vi "FaulhaberV3-Ascii_V1.vi"() -> (1 "searchnames":string[](array[string])=["devicetype", "errorregister", "pre-definederrorfield_numberoferrors", "pre-definederrorfield_standarderrorfield1", "pre-definederrorfield_standarderrorfield2", "pre-definederrorfield_standarderrorfield3", "pre-definederrorfield_standarderrorfield4", "pre-definederrorfield_standarderrorfield5", "pre-definederrorfield_standarderrorfield6", "pre-definederrorfield_standarderrorfield7", "pre-definederrorfield_standarderrorfield8", "cob-idsync", "manufacturerdevicename", "manufacturerhardwareversion", "manufacturersoftwareversion", "guardtime", "lifetimefactor", "storeparameters_numberofentries", "storeparameters_saveallparameters", "storeparameters_savecommparameters", "storeparameters_saveappparameters", "storeparameters_saveappparameters1", "storeparameters_saveappparameters2", "storeparameters_savecalparameters", "storeparameters_savefactoryparameteralls", "storeparameters_savefactoryparameterscom", "storeparameters_savefactoryparametersapp", "restoredefaultparameters_numberofentries", "restoredefaultparameters_restorealldefaultparameters", "restoredefaultparameters_restorecommdefaultparameters", "restoredefaultparameters_restoreappdefaultparameters", "restoredefaultparameters_restoreappsaved", "restoredefaultparameters_restoreapp1saved", "restoredefaultparameters_restoreapp2saved", "cob-idemcy", "consumerheartbeattime_numberofentries", "consumerheartbeattime_consumerheartbeattime", "producerheartbeattime", "identityobject_numberofentries", "identityobject_vendorid", "identityobject_productcode", "identityobject_revisionnumber", "identityobject_serialnumber", "errorbehaviour/numberoferrorclasses_numberoferrorclasses", "errorbehaviour/numberoferrorclasses_communicationerror", "serversdoparameter_numberofentries", "serversdoparameter_cob-idclienttoserver(rx)", "serversdoparameter_cob-idservertoclient(tx)", "receivepdo1parameter_numberofentries", "receivepdo1parameter_cob-idusedbyrxpdo1", "receivepdo1parameter_transmissiontype", "receivepdo2parameter_numberofentries", "receivepdo2parameter_cob-idusedbyrxpdo2", "receivepdo2parameter_transmissiontype", "receivepdo3parameters_numberofentries", "receivepdo3parameters_cob-idusedbyrxpdo3", "receivepdo3parameters_transmissiontype", "receivepdo4parameter_numberofentries", "receivepdo4parameter_cob-idusedbyrxpdo4", "receivepdo4parameter_transmissiontype", "receivepdo1mapping/numberofmappedobjects_numberofmappedobjects", "receivepdo1mapping/numberofmappedobjects_rxpdo1mappingentry1", "receivepdo1mapping/numberofmappedobjects_rxpdo1mappingentry2", "receivepdo1mapping/numberofmappedobjects_rxpdo1mappingentry3", "receivepdo1mapping/numberofmappedobjects_rxpdo1mappingentry4", "receivepdo2mapping/numberofmappedobjects_numberofmappedobjects", "receivepdo2mapping/numberofmappedobjects_rxpdo2mappingentry1", "receivepdo2mapping/numberofmappedobjects_rxpdo2mappingentry2", "receivepdo2mapping/numberofmappedobjects_rxpdo2mappingentry3", "receivepdo2mapping/numberofmappedobjects_rxpdo2mappingentry4", "receivepdo3mapping/numberofmappedobjects_numberofmappedobjects", "receivepdo3mapping/numberofmappedobjects_rxpdo3mappingentry1", "receivepdo3mapping/numberofmappedobjects_rxpdo3mappingentry2", "receivepdo3mapping/numberofmappedobjects_rxpdo3mappingentry3", "receivepdo3mapping/numberofmappedobjects_rxpdo3mappingentry4", "receivepdo4mapping/numberofmappedobjects_numberofmappedobjects", "receivepdo4mapping/numberofmappedobjects_rxpdo4mappingentry1", "receivepdo4mapping/numberofmappedobjects_rxpdo4mappingentry2", "receivepdo4mapping/numberofmappedobjects_rxpdo4mappingentry3", "receivepdo4mapping/numberofmappedobjects_rxpdo4mappingentry4", "transmitpdo1parameter_numberofentries", "transmitpdo1parameter_cob-idusedbytxpdo1", "transmitpdo1parameter_transmissiontype", "transmitpdo1parameter_eventtimer", "transmitpdo2parameter_numberofentries", "transmitpdo2parameter_cob-idusedbytxpdo2", "transmitpdo2parameter_transmissiontype", "transmitpdo2parameter_eventtimer", "transmitpdo3parameter_numberofentries", "transmitpdo3parameter_cob-idusedbytxpdo3", "transmitpdo3parameter_transmissiontype", "transmitpdo3parameter_eventtimer", "transmitpdo4parameter_numberofentries", "transmitpdo4parameter_cob-idusedbytxpdo4", "transmitpdo4parameter_transmissiontype", "transmitpdo4parameter_eventtimer", "transmitpdo1mapping/numberofmappedobjects_numberofmappedobjects", "transmitpdo1mapping/numberofmappedobjects_tpdo1mappingentry1", "transmitpdo1mapping/numberofmappedobjects_tpdo1mappingentry2", "transmitpdo1mapping/numberofmappedobjects_txpdo1mappingentry3", "transmitpdo1mapping/numberofmappedobjects_txpdo1mappingentry4", "transmitpdo2mapping/numberofmappedobjects_numberofmappedobjects", "transmitpdo2mapping/numberofmappedobjects_txpdo1mappingentry1", "transmitpdo2mapping/numberofmappedobjects_txpdo2mappingentry2", "transmitpdo2mapping/numberofmappedobjects_txpdo3mappingentry3", "transmitpdo2mapping/numberofmappedobjects_txpdo4mappingentry4", "transmitpdo3mapping/numberofmappedobjects_numberofmappedobjects", "transmitpdo3mapping/numberofmappedobjects_txpdo3mappingentry1", "transmitpdo3mapping/numberofmappedobjects_txpdo3mappingentry2", "transmitpdo3mapping/numberofmappedobjects_txpdo3mappingentry3", "transmitpdo3mapping/numberofmappedobjects_txpdo3mappingentry4", "transmitpdo4mapping/numberofmappedobjects_numberofmappedobjects", "transmitpdo4mapping/numberofmappedobjects_txpdo4mappingentry1", "transmitpdo4mapping/numberofmappedobjects_txpdo4mappingentry2", "transmitpdo4mapping/numberofmappedobjects_txpdo4mappingentry3", "transmitpdo4mapping/numberofmappedobjects_txpdo4mappingentry4", "numberofi/os_numberofentries", "numberofi/os_numberofdigitalinputs", "numberofi/os_numberofdigitaloutputs", "numberofi/os_numberofanaloginputs", "numberofi/os_numberofemulateddigitalinputs", "digitalinputsettings_numberofentries", "digitalinputsettings_selectlowerlimitswitchinputs", "digitalinputsettings_selectupperlimitswitchinputs", "digitalinputsettings_limitswitchoptioncode", "digitalinputsettings_selectreferenceswitchinput", "digitalinputsettings_emulatedinputthresholdlevel", "digitalinputsettings_selectstopinput", "digitalinputsettings_debugwritedigitalinputvalues", "digitalinputsettings_debugwritebrake/faultpin", "digitalinputsettings_selectdigitalinputsused", "digitalinputsettings_inputpolarity", "digitalinputsettings_inputthresholdlevel", "digitalinputsettings_inputfilteractive", "digitali/ostatus_numberofentries", "digitali/ostatus_digitalinputlogicalstate", "digitali/ostatus_digitalinputphysicalstate", "digitali/ostatus_digitaloutputstatus", "digitali/ostatus_writedigitaloutputs", "digitaloutputsettings_numberofentries", "digitaloutputsettings_selectfaultoutputpin", "digitaloutputsettings_selectbrakecontrolpin", "digitaloutputsettings_brakedelaytime", "digitaloutputsettings_diagout1pinselection", "digitaloutputsettings_diagout1mask", "digitaloutputsettings_diagout2pinselection", "digitaloutputsettings_diagout2mask", "digitaloutputsettings_diagout3pinselection", "digitaloutputsettings_diagout3mask", "digitaloutputsettings_diagout4pinselection", "digitaloutputsettings_diagout4mask", "digitaloutputsettings_outputpolarity", "analoginputs_numberofentries", "analoginputs_anin1gain(numerator/divisor)", "analoginputs_anin1offset", "analoginputs_anin1filtertime", "analoginputs_anin1userscaledvalue", "analoginputs_anin1resolutionasencoder", "analoginputs_anin1mininputlimit", "analoginputs_anin1maxinputlimit", "analoginputs_anin1selectdirpin", "analoginputs_anin1virtualinputvalue", "analoginputs_anin1enablevirtualinput", "analoginputs_anin2gain(numerator/divisor)", "analoginputs_anin2offset", "analoginputs_anin2filtertime", "analoginputs_anin2userscaledvalue", "analoginputs_anin2resolutionasencoder", "analoginputs_anin2mininputlimit", "analoginputs_anin2maxinputlimit", "analoginputs_anin2selectdirpin", "analoginputs_anin2virtualinputvalue", "analoginputs_anin2enablevirtualinput", "manufacturerscaledanaloginputvalues_numberofentries", "manufacturerscaledanaloginputvalues_anin1scaledvalue(ia)", "manufacturerscaledanaloginputvalues_anin2scaledvalue(ib)", "manufacturerscaledanaloginputvalues_anin3scaledvalue(ic)", "manufacturerscaledanaloginputvalues_anin4scaledvalue(halla)", "manufacturerscaledanaloginputvalues_anin5scaledvalue(hallb)", "manufacturerscaledanaloginputvalues_anin6scaledvalue(hallc)", "manufacturerscaledanaloginputvalues_anin7scaledvalue", "manufacturerscaledanaloginputvalues_anin8scaledvalue", "manufacturerscaledanaloginputvalues_anin9scaledvalue", "manufacturerscaledanaloginputvalues_anin10scaledvalue", "manufacturerscaledanaloginputvalues_anin11scaledvalue", "manufacturerscaledanaloginputvalues_anin12scaledvalue", "motorencoder_numberofentries", "motorencoder_operationmode,indexpolarity", "motorencoder_ieresolution", "motorencoder_motorencoderposition", "motorencoder_gain(numerator/divisor)", "motorencoder_motorencscaledposition", "motorencoder_absoluteencoderbits", "motorencoder_encoderstatus", "motorencoder_motorencoderactspeed", "motorencoder_speedfilter", "motorencoder_singleturnposition16bit", "referenceencoder_numberofentries", "referenceencoder_operationmode,indexpolarity", "referenceencoder_ieresolution", "referenceencoder_referenceencoderposition", "referenceencoder_gain(numerator/divisor)", "referenceencoder_refencscaledposition", "referenceencoder_referenceencoderactspeed", "referenceencoder_speedfilter", "pwminput_numberofentries", "pwminput_digitalinputpin", "pwminput_pwminputfrequency", "pwminput_dutycyclerawvalue", "pwminput_dutycyclegain(numerator/divisor)", "pwminput_dutycycleoffset", "pwminput_dutycyclescaledvalue", "pwminput_resolutionasencoder", "hallconfiguration_numberofentries", "hallconfiguration_hallsensortype", "hallconfiguration_enableadaptation", "hallconfiguration_adaptationthresholdspeed", "hallconfiguration_digitalhallsettingsofnon-faulhabermotors", "hallconfiguration_hallfilterconfiguration", "reductionratio,externalpositionencoder_numberofentries", "reductionratio,externalpositionencoder_numerator", "reductionratio,externalpositionencoder_divisor", "231f_00_numberofentries", "231f_00_231f_01", "231f_00_231f_02", "231f_00_231f_03", "231f_00_231f_04", "231f_00_231f_05", "231f_00_231f_06", "231f_00_231f_07", "231f_00_231f_08", "231f_00_231f_09", "231f_00_231f_0a", "231f_00_231f_0b", "231f_00_231f_0c", "231f_00_231f_0d", "231f_00_231f_0e", "231f_00_231f_0f", "faulhabererrorregister", "errormask_numberofentries", "errormask_emcymask", "errormask_faultmask", "errormask_erroroutmask", "errormask_disablevoltagemaskmanufacturer", "errormask_disablevoltagemaskuser", "errormask_quickstopmask", "errormask_errorbitmask", "errorcodes_numberofentries", "errorcodes_scriptingerror", "devicestatus_numberofentries", "devicestatus_devicestatusword", "devicestatus_limitcheckdelaytime", "devicestatus_reserved3", "devicestatus_reserved4", "devicestatus_reserved5", "devicestatus_reserved6", "devicestatus_reserved7", "devicestatus_reserved8", "devicestatus_reserved9", "voltagemonitor_numberofentries", "voltagemonitor_devicesupplylowerthreshold", "voltagemonitor_motorsupplylowerthreshold", "voltagemonitor_motorsupplymaxthreshold", "voltagemonitor_motorsupplyupperthreshold", "voltagemonitor_voltageerrordelaytime", "voltagemonitor_devicesupplyvoltage", "voltagemonitor_motorsupplyvoltage", "devicetemperature_numberofentries", "devicetemperature_cputemperature", "devicetemperature_powerstagetemperature", "devicetemperature_windingtemperature", "devicetemperature_cputemperatureshutdownthreshold", "devicetemperature_cputemperaturewarningthreshold", "devicetemperature_powerstagetemperatureshutdownthreshold", "devicetemperature_powerstagetemperaturewarningthreshold", "devicetemperature_windingtemperatureshutdownthreshold", "devicetemperature_windingtemperaturewarningthreshold", "devicetemperature_motorntctemperature", "devicetemperature_motorntcenable", "devicedata_numberofentries", "devicedata_devicenominalcurrent", "devicedata_devicepeakcurrent", "devicedata_devicenominalvoltage", "devicedataforthermalmodel_numberofentries", "devicedataforthermalmodel_controllertype", "devicedataforthermalmodel_powerstagerdson", "devicedataforthermalmodel_powerstagelossfactor", "devicedataforthermalmodel_powerstagerth1", "devicedataforthermalmodel_powerstagetimeconstant1", "devicedataforthermalmodel_powerstagerth2", "devicedataforthermalmodel_powerstagetimeconstant2", "devicedataforthermalmodel_powerstagerth3", "devicedataforthermalmodel_powerstagerth4", "motorandapplicationdataformotorcontrol_numberofentries", "motorandapplicationdataformotorcontrol_ratedcurrent", "motorandapplicationdataformotorcontrol_continouscurrent", "motorandapplicationdataformotorcontrol_peakcurrent", "motorandapplicationdataformotorcontrol_torqueconstant/forceconstant", "motorandapplicationdataformotorcontrol_terminalinductance", "motorandapplicationdataformotorcontrol_inductanceld", "motorandapplicationdataformotorcontrol_numberofpolepairs", "motorandapplicationdataformotorcontrol_phaseangleoffset", "motorandapplicationdataformotorcontrol_rotorinertia/rodweight", "motorandapplicationdataformotorcontrol_loadinertia/loadmass", "motorandapplicationdataformotorcontrol_motortype", "motorandapplicationdataformotorcontrol_magneticpitchoflinearmotor", "motorandapplicationdataformotorcontrol_filterphaseinductance", "motorandapplicationdataformotorcontrol_factorspeedconstant", "motorandapplicationdataformotorcontrol_stepsperturn", "motorandapplicationdataformotorcontrol_stepperinterpolationfactor", "motorandapplicationdataformotorcontrol_steppercurrentreductionatn=0", "motorandapplicationdataformotorcontrol_currentholdingtimeatn=0", "motorandapplicationdataforthermalmotormodel_numberofentries", "motorandapplicationdataforthermalmotormodel_terminalresistance", "motorandapplicationdataforthermalmotormodel_friction", "motorandapplicationdataforthermalmotormodel_friction,dynamic", "motorandapplicationdataforthermalmotormodel_thermalresistance1", "motorandapplicationdataforthermalmotormodel_thermalresistance2", "motorandapplicationdataforthermalmotormodel_thermaltimeconstant1", "motorandapplicationdataforthermalmotormodel_thermaltimeconstant2", "motorandapplicationdataforthermalmotormodel_ambienttemperature", "motorandapplicationdataforthermalmotormodel_reductionofthermalresistance2", "motorandapplicationdataforthermalmotormodel_selectionofthermalmodel", "motoralignmentparameters_numberofentries", "motoralignmentparameters_setuptime", "motoralignmentparameters_deltatimestep1", "motoralignmentparameters_deltatimestep2", "motoralignmentparameters_deltatimestep3", "motoralignmentparameters_deltapostiontolerance", "motoralignmentresults_numberofentries", "motoralignmentresults_positiona1", "motoralignmentresults_positionb", "motoralignmentresults_positiona2", "switchpositionforactualvalues_numberofentries", "switchpositionforactualvalues_actualcommutationanglesource", "switchpositionforactualvalues_actualvelocitysource", "switchpositionforactualvalues_actualpositionsource", "discretesources_numberofentries", "discretesources_targetvoltagesource", "discretesources_targetcurrentsource", "discretesources_targetvelocitysource", "discretesources_targetpositionsource", "cyclicmodeinterpolationrate", "manufacturerspecifiedbits_numberofentries", "manufacturerspecifiedbits_bitmaskforbit14", "manufacturerspecifiedbits_bitmaskforbit15", "selectionofcontrollerscaling", "operationmodeoptions", "generalparameters_numberofentries", "generalparameters_commutationtype", "generalparameters_motoroutputvoltagedc", "generalparameters_motoroutputvoltageblblock", "generalparameters_motoroutputvoltagexd", "generalparameters_motoroutputvoltagexq", "generalparameters_sinusoutputvoltageua", "generalparameters_sinusoutputvoltageub", "generalparameters_sinusoutputvoltageuc", "generalparameters_sinusoutputvoltageud", "targetvoltage", "torquecontrolparameters_numberofentries", "torquecontrolparameters_gainkpi", "torquecontrolparameters_integraltimetni", "fluxcontrolparameters_numberofentries", "fluxcontrolparameters_gainkpi", "fluxcontrolparameters_integraltimetni", "velocitycontrolparameters_numberofentries", "velocitycontrolparameters_gainkp", "velocitycontrolparameters_integraltimetn", "velocitycontrolparameters_velocitydeviationthreshold", "velocitycontrolparameters_velocitydeviationtime", "velocitycontrolparameters_velocitywarningthreshold", "velocitycontrolparameters_integralpartoption", "velocityfilterparameters_numberofentries", "velocityfilterparameters_actualvelocityfiltertf", "velocityfilterparameters_displayvelocityfilter", "setpointvelocityfilterparameters_numberofentries", "setpointvelocityfilterparameters_setpointvelocityfiltertf", "setpointvelocityfilterparameters_setpointfilterenable", "gainscheduling_numberofentries", "gainscheduling_gainfactorkpn", "gainscheduling_gainfactorkv", "positioncontrolparameters_numberofentries", "positioncontrolparameters_gainkv", "currentfeedforwardparameters_numberofentries", "currentfeedforwardparameters_currentfeedforwardfactor", "currentfeedforwardparameters_currentfeedforwarddelay", "velocityfeedforwardparameters_numberofentries", "velocityfeedforwardparameters_velocityfeedforwardfactor", "velocityfeedforwardparameters_velocityfeedforwarddelay", "currentfilterparameters_numberofentries", "currentfilterparameters_displaycurrentfiltertf", "currentfilterparameters_displaytorquefiltertf", "currentcompensationparameters_numberofentries", "currentcompensationparameters_gravitycompensation", "currentcompensationparameters_positivefrictioncompensation", "currentcompensationparameters_negativefrictioncompensation", "positivetorquelimithoming", "negativetorquelimithoming", "actualvalues_numberofentries", "actualvalues_motorcurrentidactualvalue", "actualvalues_motorcurrentiqactualvalue", "actualvalues_motorcurrrentiblockactualvalue", "actualvalues_motorcurrentidcactualvalue", "actualvalues_velocityactualinternalvalue", "actualvalues_positionactualinternalvalue", "actualvalues_actualcommutationsegment", "actualvalues_actualcommutationangle", "actualvalues_reserved9", "actualvalues_reserved10", "traceconfiguration_numberofentries", "traceconfiguration_triggervalue", "traceconfiguration_triggerthreshold", "traceconfiguration_triggeroffset", "traceconfiguration_triggermode", "traceconfiguration_bufferlength", "traceconfiguration_sampletime", "traceconfiguration_tracesourceofchannel1", "traceconfiguration_tracesourceofchannel2", "traceconfiguration_tracesourceofchannel3", "traceconfiguration_tracesourceofchannel4", "traceconfiguration_monitorsourceofchannel1", "traceconfiguration_monitorsourceofchannel2", "traceconfiguration_monitorsourceofchannel3", "traceconfiguration_monitorsourceofchannel4", "traceconfiguration_extendedrecordermode", "tracebuffer_numberofentries", "tracebuffer_tracestate", "logictriggerconfiguration_numberofentries", "logictriggerconfiguration_logictriggerandmask", "logictriggerconfiguration_logictriggerormask", "eventtriggerconfiguration_numberofentries", "eventtriggerconfiguration_eventtriggereventselection", "eventflagconfiguration_numberofentries", "eventflagconfiguration_eventflagsetmask", "eventflagconfiguration_eventflagresetmask", "tracechannelconfiguration_numberofentries", "tracechannelconfiguration_channel1filtertime", "tracechannelconfiguration_channel1sampletime", "tracechannelconfiguration_channel1numberofsamples", "tracechannelconfiguration_channel1monitoringvalues", "tracechannelconfiguration_channel1starteventselection", "tracechannelconfiguration_channel1updateeventselection", "tracechannelconfiguration_channel1numberofeval-cycles", "tracechannelconfiguration_channel1numberofturnovers", "tracechannelconfiguration_channel1done", "tracechannelconfiguration_channel1absminvalue", "tracechannelconfiguration_channel1absmaxvalue", "tracechannelconfiguration_channel1minimum", "tracechannelconfiguration_channel1maximum", "tracechannelconfiguration_channel1meanvalue", "tracechannelconfiguration_channel1rmsvalue", "tracechannelconfiguration_channel1periodtime", "tracechannelconfiguration_channel1sigma", "tracechannelconfiguration_numberofentries", "tracechannelconfiguration_channel2filtertime", "tracechannelconfiguration_channel2sampletime", "tracechannelconfiguration_channel2numberofsamples", "tracechannelconfiguration_channel2monitoringvalues", "tracechannelconfiguration_channel2starteventselection", "tracechannelconfiguration_channel2updateeventselection", "tracechannelconfiguration_channel2numberofeval-cycles", "tracechannelconfiguration_channel2numberofturn-overs", "tracechannelconfiguration_channel2done", "tracechannelconfiguration_channel2absminvalue", "tracechannelconfiguration_channel2absmaxvalue", "tracechannelconfiguration_channel2minimum", "tracechannelconfiguration_channel2maximum", "tracechannelconfiguration_channel2meanvalue", "tracechannelconfiguration_channel2rmsvalue", "tracechannelconfiguration_channel2periodtime", "tracechannelconfiguration_channel2sigma", "tracechannelconfiguration_numberofentries", "tracechannelconfiguration_channel3filtertime", "tracechannelconfiguration_channel3sampletime", "tracechannelconfiguration_channel3numberofsamples", "tracechannelconfiguration_channel3monitoringvalues", "tracechannelconfiguration_channel3starteventselection", "tracechannelconfiguration_channel3updateeventselection", "tracechannelconfiguration_channel3numberofeval-cycles", "tracechannelconfiguration_channel3numberofturn-overs", "tracechannelconfiguration_channel3done", "tracechannelconfiguration_channel3absminvalue", "tracechannelconfiguration_channel3absmaxvalue", "tracechannelconfiguration_channel3minimum", "tracechannelconfiguration_channel3maximum", "tracechannelconfiguration_channel3meanvalue", "tracechannelconfiguration_channel3rmsvalue", "tracechannelconfiguration_channel3periodtime", "tracechannelconfiguration_channel3sigma", "tracechannelconfiguration_numberofentries", "tracechannelconfiguration_channel4filtertime", "tracechannelconfiguration_channel4sampletime", "tracechannelconfiguration_channel4numberofsamples", "tracechannelconfiguration_channel4monitoringvalues", "tracechannelconfiguration_channel4starteventselection", "tracechannelconfiguration_channel4updateeventselection", "tracechannelconfiguration_channel4numberofeval-cycles", "tracechannelconfiguration_channel4numberofturn-overs", "tracechannelconfiguration_channel4done", "tracechannelconfiguration_channel4absminvalue", "tracechannelconfiguration_channel4absmaxvalue", "tracechannelconfiguration_channel4minimum", "tracechannelconfiguration_channel4maximum", "tracechannelconfiguration_channel4meanvalue", "tracechannelconfiguration_channel4rmsvalue", "tracechannelconfiguration_channel4periodtime", "tracechannelconfiguration_channel4sigma", "prbsgenerator_numberofentries", "prbsgenerator_shiftregisterinit", "prbsgenerator_gain", "prbsgenerator_offset", "prbsgenerator_sampleratefactor", "prbsgenerator_enable", "startupgenerator_numberofentries", "startupgenerator_speedthreshold", "startupgenerator_timeouttime", "startupgenerator_targetvalue", "startupgenerator_reset", "startupgenerator_enable", "startupgenerator_ready", "startupgenerator_timethreshold", "startupgenerator_iteration", "sinusoidalexcitation_numberofentries", "sinusoidalexcitation_amplitude", "sinusoidalexcitation_frequency", "sinusoidalexcitation_enable", "selectsignalgeneratorsource_numberofentries", "selectsignalgeneratorsource_selector", "23f0_00_numberofentries", "23f0_00_23f0_01", "23f0_00_23f0_02", "23f0_00_23f0_03", "23f0_00_23f0_04", "23f0_00_23f0_05", "23f0_00_23f0_06", "23f1_00_numberofentries", "23f1_00_23f1_01", "23f1_00_23f1_02", "23f2_00_numberofentries", "23f2_00_actualstate", "23f2_00_demandposition", "23f2_00_demandspeed", "23f2_00_demandacceleration", "23f2_00_initialstate", "communicationparameters_numberofentries", "communicationparameters_canrate", "communicationparameters_rs232rate", "communicationparameters_nodeid", "communicationparameters_communicationsettings", "communicationparameters_rs232netmode", "communicationparameters_comstate", "communicationparameters_errstate", "usbdelay", "faid", "bootloaderswversion", "odrevisionnumber", "swrevisionnumber", "xdcnumber", "calaccess_numberofentries", "calaccess_calkey", "adcscaling(offset|gain)_numberofentries", "adcscaling(offset|gain)_iascaling", "adcscaling(offset|gain)_ibscaling", "adcscaling(offset|gain)_icscaling", "adcscaling(offset|gain)_hallascaling", "adcscaling(offset|gain)_hallbscaling", "adcscaling(offset|gain)_hallcscaling", "adcscaling(offset|gain)_analoginput1scaling", "adcscaling(offset|gain)_analoginput2scaling", "adcscaling(offset|gain)_uelscaling", "adcscaling(offset|gain)_udcscaling", "adcscaling(offset|gain)_internaltemperaturescaling", "adcscaling(offset|gain)_externaltemperaturescaling", "adcscaling(offset|gain)_motorntcgain", "adcscaling(offset|gain)_motorntcoffset", "hallscaling_numberofentries", "hallscaling_gaina", "hallscaling_hallaoffset", "hallscaling_hallasin", "hallscaling_hallacos", "hallscaling_corra", "hallscaling_hallboffset", "hallscaling_hallbsin", "hallscaling_hallbcos", "hallscaling_corrb", "hallscaling_hallcoffset", "hallscaling_hallcsin", "hallscaling_hallccos", "hallscaling_offseta", "hallscaling_offsetb", "internalfilterparameters_numberofentries", "internalfilterparameters_filtertimeactualvelocity", "internalfilterparameters_filtertimeia", "internalfilterparameters_filtertimeib", "internalfilterparameters_filtertimeic", "internalfilterparameters_filtertimeuel", "internalfilterparameters_filtertimeumot", "internalfilterparameters_additionalfiltertimeuel", "internalfilterparameters_additionalfiltertimeumot", "internalfilterparameters_filtertimeiqthermalmodel", "internalfilterparameters_filtertimeidthermalmodel", "internalfilterparameters_filtertimeimotthermalmodel", "internalfilterparameters_filtertimesetpointvoltagemodel", "internalfilterparameters_filtertimeelectricaltimeconstant", "bootoptions", "hallcompensation_numberofentries", "hallcompensation_entry01", "hallcompensation_entry02", "hallcompensation_entry03", "hallcompensation_entry04", "hallcompensation_entry05", "hallcompensation_entry06", "hallcompensation_entry07", "hallcompensation_entry08", "hallcompensation_entry09", "hallcompensation_entry10", "hallcompensation_entry11", "hallcompensation_entry12", "encodercompensation_numberofentries", "encodercompensation_value0", "encodercompensation_value1", "encodercompensation_value2", "encodercompensation_value3", "encodercompensation_value4", "encodercompensation_value5", "encodercompensation_value6", "encodercompensation_value7", "encodercompensation_value8", "encodercompensation_value9", "encodercompensation_value10", "encodercompensation_value11", "encodercompensation_value12", "encodercompensation_value13", "encodercompensation_value14", "encodercompensation_value15", "encodercompensation_value16", "encodercompensation_value17", "encodercompensation_value18", "encodercompensation_value19", "encodercompensation_value20", "encodercompensation_value21", "encodercompensation_value22", "encodercompensation_value23", "encodercompensation_value24", "encodercompensation_value25", "encodercompensation_value26", "encodercompensation_value27", "encodercompensation_value28", "encodercompensation_value29", "encodercompensation_value30", "encodercompensation_value31", "encodercompensation_value32", "encodercompensation_value33", "encodercompensation_value34", "encodercompensation_value35", "encodercompensation_value36", "encodercompensation_value37", "encodercompensation_value38", "encodercompensation_value39", "encodercompensation_value40", "encodercompensation_value41", "encodercompensation_value42", "encodercompensation_value43", "encodercompensation_value44", "encodercompensation_value45", "encodercompensation_value46", "encodercompensation_value47", "encodercompensation_value48", "encodercompensation_value49", "encodercompensation_value50", "encodercompensation_value51", "encodercompensation_value52", "encodercompensation_value53", "encodercompensation_value54", "encodercompensation_value55", "encodercompensation_value56", "encodercompensation_value57", "encodercompensation_value58", "encodercompensation_value59", "encodercompensation_value60", "encodercompensation_value61", "encodercompensation_value62", "encodercompensation_value63", "pwmfrequency", "250f_00", "drivesystemgear_numberofentries", "drivesystemgear_gearrationum", "drivesystemgear_gearratioden", "drivesystemloadtransmission_numberofentries", "drivesystemloadtransmission_loadtransmission", "drivesystemloadtransmission_loadtransmissionrationum", "drivesystemloadtransmission_loadtransmissionratioden", "drivesystemnumbers_numberofentries", "drivesystemnumbers_gearcatalognumber", "drivesystemnumbers_encodercatalogenumber", "drivesystemnumbers_drivecombinationnumber", "drivesystemunits_numberofentries", "drivesystemunits_unitreference", "drivesystemunits_unitnames", "nominalvoltage", "drivesystemsettings", "oemdevicedata_numberofentries", "oemdevicedata_oemproductdescriptor", "oemdevicedata_oemproductcode", "oemdevicedata_oemserialnumber", "userprograms_numberofentries", "userprograms_userprogram1startaddress", "userprograms_userprogram2startaddress", "userprograms_userprogram3startaddress", "userprograms_userprogram4startaddress", "userprograms_userprogram5startaddress", "userprograms_userprogram6startaddress", "userprograms_userprogram7startaddress", "userprograms_userprogram8startaddress", "activeprogram_numberofentries", "activeprogram_actualprogramcommand", "activeprogram_actualprogramnumber", "activeprogram_actualprogramposition", "activeprogram_actualprogramstate", "activeprogram_breakpointaddress", "activeprogram_upload/downloadbuffer", "activeprogram_errorstate", "activeprogram_errorcode", "activeprogram_programmemory", "autostartprogram", "accesskey", "debuguserprogram_numberofentries", "debuguserprogram_selectvariable", "debuguserprogram_selectedvariablevalue", "userprogramvariables_numberofentries", "userprogramvariables_userprogvariablea", "userprogramvariables_userprogvariableb", "userprogramvariables_userprogvariablec", "userprogramvariables_userprogvariabled", "userprogramvariables_userprogvariablee", "userprogramvariables_userprogvariablef", "userprogramvariables_userprogvariableg", "userprogramvariables_userprogvariableh", "userprogramvariables_userprogvariablei", "userprogramvariables_userprogvariablej", "userprogramvariables_userprogvariablek", "userprogramvariables_userprogvariablel", "userprogramvariables_userprogvariablem", "userprogramvariables_userprogvariablen", "userprogramvariables_userprogvariableo", "userprogramvariables_userprogvariablep", "userprogramvariables_userprogvariableq", "userprogramvariables_userprogvariabler", "userprogramvariables_userprogvariables", "userprogramvariables_userprogvariablet", "userprogramvariables_userprogvariableu", "userprogramvariables_userprogvariablev", "userprogramvariables_userprogvariablew", "userprogramvariables_userprogvariablex", "userprogramvariables_userprogvariabley", "userprogramvariables_userprogvariablez", "scriptingstack/numberoflevels_numberoflevels", "scriptingstack/numberoflevels_callstacklevel0", "scriptingstack/numberoflevels_callstacklevel1", "scriptingstack/numberoflevels_callstacklevel2", "scriptingstack/numberoflevels_callstacklevel3", "scriptingstack/numberoflevels_callstacklevel4", "scriptingstack/numberoflevels_callstacklevel5", "scriptingstack/numberoflevels_callstacklevel6", "scriptingstack/numberoflevels_callstacklevel7", "scriptingstack/numberoflevels_callstacklevel8", "scriptingstack/numberoflevels_callstacklevel9", "scriptingstack/numberoflevels_callstacklevel10", "scriptingstack/numberoflevels_callstacklevel11", "scriptingstack/numberoflevels_callstacklevel12", "scriptingstack/numberoflevels_callstacklevel13", "scriptingstack/numberoflevels_callstacklevel14", "variableaccesskey", "programconstants_numberofentries", "programconstants_programconstant0", "programconstants_programconstant1", "programconstants_programconstant2", "programconstants_programconstant3", "programconstants_programconstant4", "programconstants_programconstant5", "programconstants_programconstant6", "programconstants_programconstant7", "programconstants_programconstant8", "programconstants_programconstant9", "programconstants_programconstant10", "programconstants_programconstant11", "programconstants_programconstant12", "programconstants_programconstant13", "programconstants_programconstant14", "programconstants_programconstant15", "abortconnectionoptioncode", "controlword", "statusword", "quick-stopoptioncode", "shutdownoptioncode", "disableoperationoptioncode", "haltoptioncode", "faultreactionoptioncode", "modesofoperation", "modesofoperationdisplay", "positiondemandvalue", "positionactualinternalvalue", "positionactualvalue", "followingerrorwindow", "followingerrortimeout", "positionwindow", "positionwindowtime", "velocitydemandvalue", "velocityactualvalue", "velocitywindow", "velocitywindowtime", "velocitythreshold", "velocitythresholdtime", "targettorque", "maxtorque", "torquedemand", "torqueactualvalue", "currentactualvalue", "targetposition", "positionrangelimit_numberofentries", "positionrangelimit_minpositionrangelimit", "positionrangelimit_maxpositionrangelimit", "homeoffset", "softwarepositionlimit_numberofentries", "softwarepositionlimit_minpositionlimit", "softwarepositionlimit_maxpositionlimit", "polarity", "maxmotorspeed", "profilevelocity", "profileacceleration", "profiledeceleration", "quickstopdeceleration", "motionprofiletype", "positionencoderresolution_numberofentries", "positionencoderresolution_encoderincrements", "positionencoderresolution_motorrevolutions", "velocityencoderresolution_numberofentries", "velocityencoderresolution_encoderincrements", "velocityencoderresolution_motorrevolutions", "gearratio_numberofentries", "gearratio_motorshaftrevolutions", "gearratio_drivingshaftrevolutions", "feedconstant_numberofentries", "feedconstant_feed", "feedconstant_shaftrevolutions", "velocityfactor_numberofentries", "velocityfactor_numerator", "velocityfactor_divisor", "homingmethod", "homingspeeds_numberofentries", "homingspeeds_switchseekvelocity", "homingspeeds_homingspeed", "homingacceleration", "positionoffset", "velocityoffset", "torqueoffset", "touchprobefunction", "touchprobestatus", "touchprobe1positiveedge", "touchprobe1negativeedge", "touchprobe2positiveedge", "touchprobe2negativeedge", "maxacceleration", "maxdeceleration", "touchprobe1positiveedgecounter", "touchprobe1negativeedgecounter", "touchprobe2positiveedgecounter", "touchprobe2negativeedgecounter", "positivetorquelimitvalue", "negativetorquelimitvalue", "positionoptioncode", "followingerroractualvalue", "digitalinputs", "targetvelocity", "motorcataloguenumber", "supporteddrivemodes", "drivecataloguenumber"], 2 "ID":u32[](array[numeric])=[268435456, 268500992, 268632064, 268632065, 268632066, 268632067, 268632068, 268632069, 268632070, 268632071, 268632072, 268763136, 268959744, 269025280, 269090816, 269221888, 269287424, 269484032, 269484033, 269484034, 269484035, 269484036, 269484037, 269484038, 269484039, 269484040, 269484041, 269549568, 269549569, 269549570, 269549571, 269549572, 269549573, 269549574, 269746176, 269877248, 269877249, 269942784, 270008320, 270008321, 270008322, 270008323, 270008324, 271122432, 271122433, 301989888, 301989889, 301989890, 335544320, 335544321, 335544322, 335609856, 335609857, 335609858, 335675392, 335675393, 335675394, 335740928, 335740929, 335740930, 369098752, 369098753, 369098754, 369098755, 369098756, 369164288, 369164289, 369164290, 369164291, 369164292, 369229824, 369229825, 369229826, 369229827, 369229828, 369295360, 369295361, 369295362, 369295363, 369295364, 402653184, 402653185, 402653186, 402653189, 402718720, 402718721, 402718722, 402718725, 402784256, 402784257, 402784258, 402784261, 402849792, 402849793, 402849794, 402849797, 436207616, 436207617, 436207618, 436207619, 436207620, 436273152, 436273153, 436273154, 436273155, 436273156, 436338688, 436338689, 436338690, 436338691, 436338692, 436404224, 436404225, 436404226, 436404227, 436404228, 587202560, 587202561, 587202562, 587202563, 587202564, 588251136, 588251137, 588251138, 588251139, 588251140, 588251141, 588251142, 588251144, 588251145, 588251151, 588251152, 588251153, 588251154, 588316672, 588316673, 588316674, 588316675, 588316676, 588382208, 588382209, 588382210, 588382211, 588382216, 588382217, 588382218, 588382219, 588382220, 588382221, 588382222, 588382223, 588382224, 588447744, 588447745, 588447746, 588447747, 588447748, 588447749, 588447750, 588447751, 588447752, 588447753, 588447754, 588447761, 588447762, 588447763, 588447764, 588447765, 588447766, 588447767, 588447768, 588447769, 588447770, 588513280, 588513281, 588513282, 588513283, 588513284, 588513285, 588513286, 588513287, 588513288, 588513289, 588513290, 588513291, 588513292, 588578816, 588578817, 588578818, 588578819, 588578820, 588578821, 588578822, 588578823, 588578824, 588578825, 588578826, 588644352, 588644353, 588644354, 588644355, 588644356, 588644357, 588644360, 588644361, 588709888, 588709889, 588709890, 588709891, 588709892, 588709893, 588709894, 588709895, 588775424, 588775425, 588775426, 588775427, 588775428, 588775429, 588840960, 588840961, 588840962, 589234176, 589234177, 589234178, 589234179, 589234180, 589234181, 589234182, 589234183, 589234184, 589234185, 589234186, 589234187, 589234188, 589234189, 589234190, 589234191, 589299712, 589365248, 589365249, 589365250, 589365251, 589365252, 589365253, 589365254, 589365255, 589430784, 589430785, 589561856, 589561857, 589561858, 589561859, 589561860, 589561861, 589561862, 589561863, 589561864, 589561865, 589627392, 589627393, 589627394, 589627395, 589627396, 589627397, 589627398, 589627399, 589692928, 589692929, 589692930, 589692931, 589692932, 589692933, 589692934, 589692935, 589692936, 589692937, 589692938, 589692939, 589758464, 589758465, 589758466, 589758467, 589824000, 589824001, 589824002, 589824003, 589824004, 589824005, 589824006, 589824007, 589824008, 589824009, 589889536, 589889537, 589889538, 589889539, 589889540, 589889541, 589889542, 589889543, 589889544, 589889545, 589889546, 589889547, 589889548, 589889549, 589889550, 589889551, 589889552, 589889553, 589889554, 589955072, 589955073, 589955074, 589955075, 589955076, 589955077, 589955078, 589955079, 589955080, 589955081, 589955082, 590020608, 590020609, 590020610, 590020611, 590020612, 590020613, 590086144, 590086145, 590086146, 590086147, 590348288, 590348289, 590348290, 590348291, 590413824, 590413825, 590413826, 590413827, 590413828, 590479360, 591003648, 591003649, 591003650, 591265792, 591331328, 591396864, 591396865, 591396866, 591396867, 591396868, 591396869, 591396870, 591396871, 591396872, 591396873, 591462400, 591527936, 591527937, 591527938, 591593472, 591593473, 591593474, 591659008, 591659009, 591659010, 591659011, 591659012, 591659013, 591659014, 591724544, 591724545, 591724546, 591790080, 591790081, 591790082, 591855616, 591855617, 591855618, 591921152, 591921153, 591986688, 591986689, 591986690, 592052224, 592052225, 592052226, 592117760, 592117761, 592117762, 592183296, 592183297, 592183298, 592183299, 592445440, 592510976, 593494016, 593494017, 593494018, 593494019, 593494020, 593494021, 593494022, 593494023, 593494024, 593494025, 593494026, 594542592, 594542593, 594542594, 594542595, 594542596, 594542597, 594542598, 594542599, 594542600, 594542601, 594542602, 594542603, 594542604, 594542605, 594542606, 594542607, 594608128, 594608129, 594673664, 594673665, 594673666, 594739200, 594739201, 594804736, 594804737, 594804738, 595066880, 595066881, 595066882, 595066883, 595066884, 595066885, 595066886, 595066887, 595066894, 595066895, 595066896, 595066897, 595066898, 595066899, 595066900, 595066901, 595066902, 595066903, 595132416, 595132417, 595132418, 595132419, 595132420, 595132421, 595132422, 595132423, 595132430,
